vi "Extract_DATA_ID_from_header.vi"() -> ()   [LabVIEW 2016]
uses:
  <vilib>/regexp/Match Regular Expression.xnode
panel:
  out "array":string[](array[string])
  out "Array":i32[](array[numeric])
  in  "Size":i32=25
  out "Array 4":string[](array[string])
  out "Array 3":string[](array[string])
  out "offset past match":i32
  out "error out":errorcluster
  out "text":string
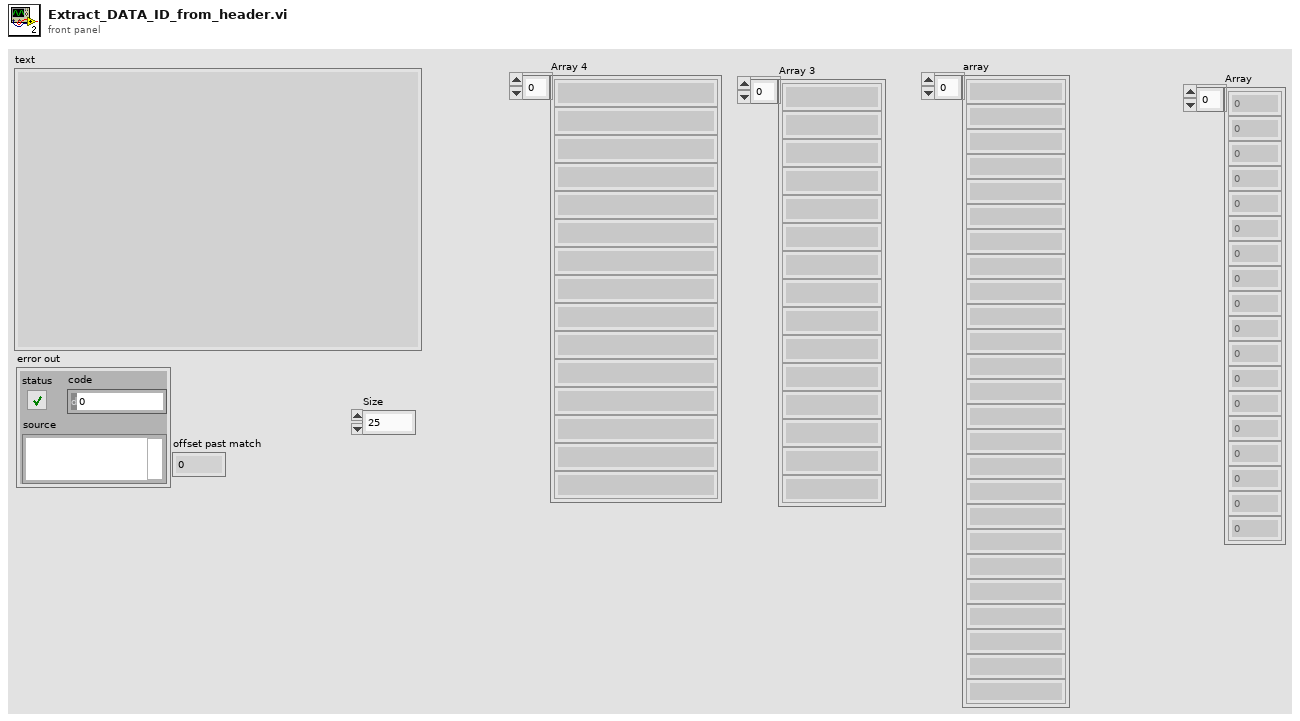
[diagram p1: front panel]
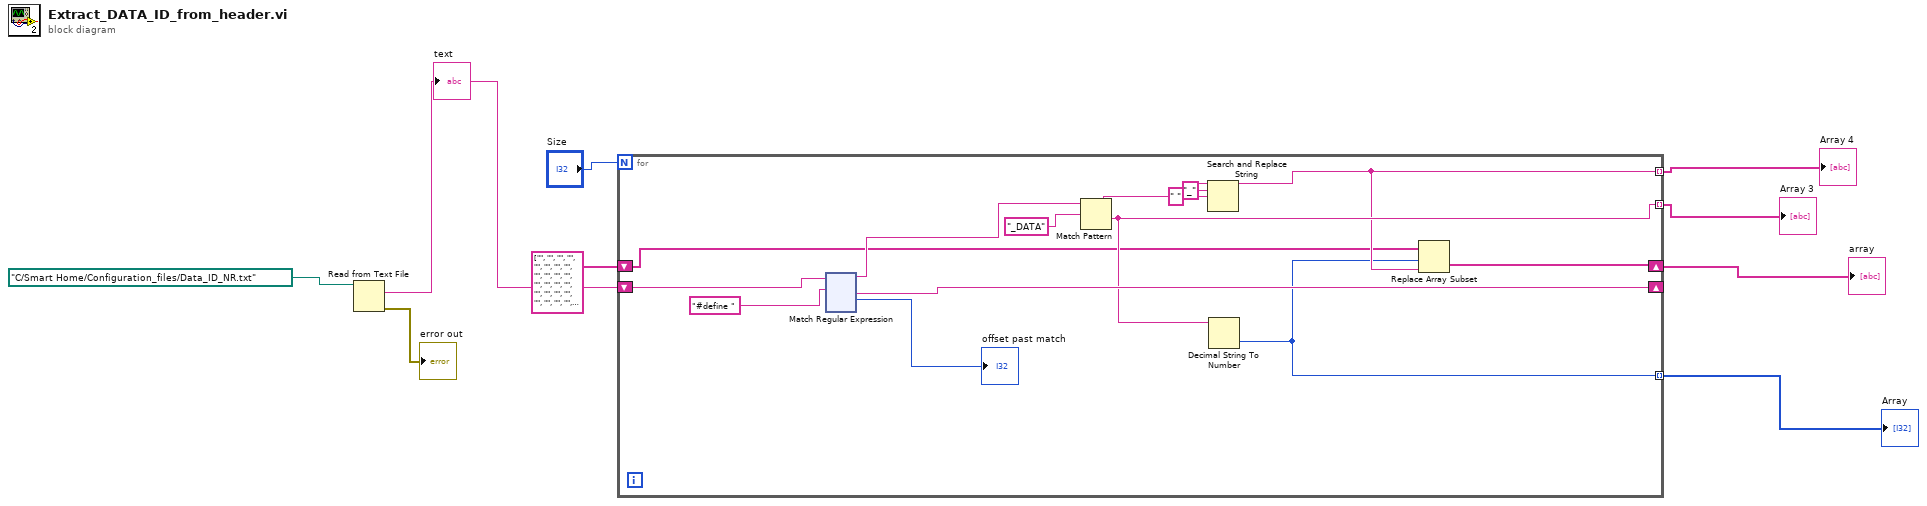
[diagram p0: block diagram]
diagram:
  n1 = Read from Text File(file (use dialog)=path "C:/Smart Home/Configuration_files/Data_ID_NR.txt") -> (text=w7:string, error out=→"error out":errorcluster)  [unwired: 3 in, 2 out]
  "text" <- w7
  n2 = for {
    N: "Size" -> [_]
    shift-right: [w21] -> _
    shift-left: w7 -> [w23]
    tunnel: [w14] -> w5 mode=indexing
    tunnel: [w13] -> w4 mode=indexing
    tunnel: [w12] -> w3 mode=indexing
    shift-right: [w11] -> w1
    shift-left: string[] ["", "", "", "", "", "", "", "", "", "", "", "", "", "", "", "", "", "", "", "", "", "", "", "", "", "", "", "", "", "", "0"] ("array") -> [w10]
    n3 = xnode "Match Regular Expression"("input string"=w23, "regular expression"="#define ") -> ("before match"=w19:string, "after match"=w21:string, "offset past match"=→"offset past match":i32)  [unwired: 4 in, 2 out]
    n4 = Match Pattern(string=w19, regular expression="_DATA" ("format string")) -> (before substring=w17:string, after substring=w14:string)  [unwired: 1 in, 2 out]
    n5 = Search and Replace String(input string=w17, search string="_", replace string=" " ("replace string (\"\")")) -> (result string=w13:string)  [unwired: 5 in, 3 out]
    n6 = Decimal String To Number(string=w14) -> (number=w12:i32)  [unwired: 2 in, 1 out]
    n7 = Replace Array Subset(array=w10, new element=w13, index=w12) -> (w11:string[])
  }
  "Array 3" <- w5
  "Array 4" <- w4
  "Array" <- w3
  "array" <- w1
